vi "Capture and save.vi"() -> ()   [LabVIEW 2023]
uses:
  <vilib>/userDefined/High Color/IMAQdx.ctl
  <vilib>/vision/driver/NI_Vision_Acquisition_Software.lvlib
panel:
  in  "Stop Button":bool
  in  "Save":bool
  out "Appended Path":path
  in  "File Path 2":path
  out "Image":T1(plugin-control)
  in  "Session In":T2
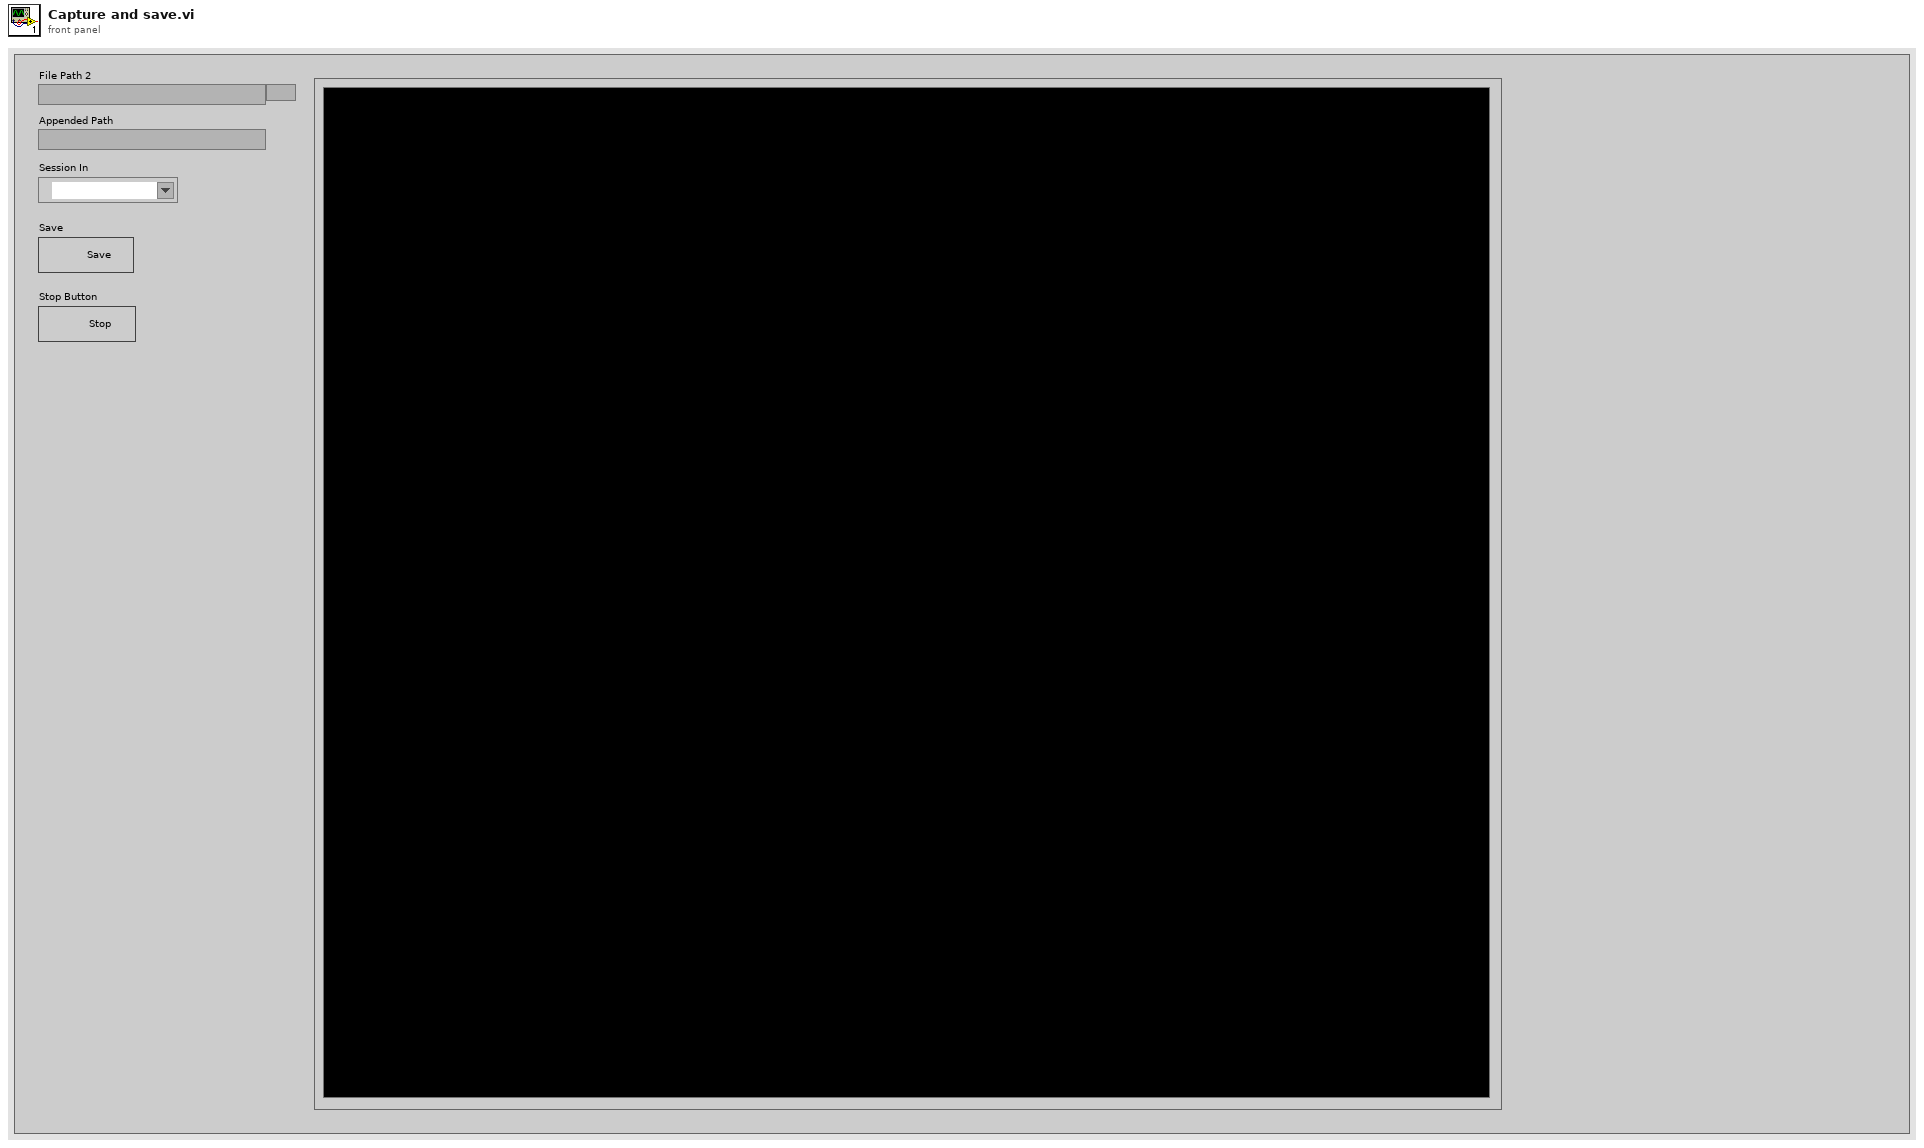
[diagram p1: front panel]
types:
  T1 = typedef "IMAQ Image.ctl" = refnum<image>
  T2 = typedef "IMAQdx.ctl" = refnum<k21>
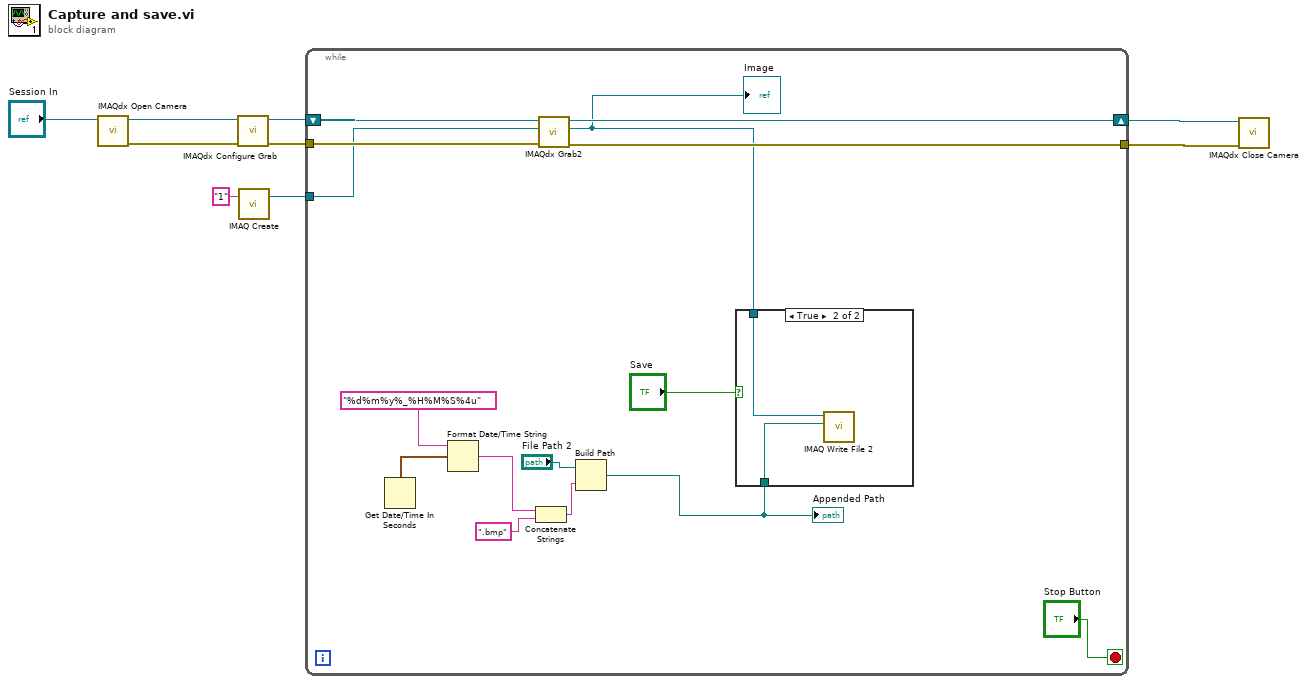
[diagram p0: block diagram]
diagram:
  n1 = call <vilib>:"IMAQdx Open Camera.vi"("Session In"="Session In") -> ("error out"=w8:errorcluster, "Session Out"=w3:T2)  [unwired: 9 in]
  n2 = call <vilib>:"IMAQdx Configure Grab.vi"("error in"=w8, "Session In"=w3) -> ("error out"=w1:errorcluster, "Session Out"=w2:T2)  [unwired: 8 in]
  n3 = call "IMAQ Create"("Image Name"="1") -> ("New Image"=w4:T1)  [unwired: 4 in, 1 out]
  n4 = while {
    shift-right: [w21] -> w7
    shift-left: w2 -> [w24]
    tunnel: w1 -> [w23]
    tunnel: [w22] -> w6
    tunnel: w4 -> [w20]
    stop <- "Stop Button" stop-if-true
    n5 = Get Date/Time In Seconds() -> (seconds since 1Jan1904=w18:timestamp)
    n6 = Format Date/Time String(time format string (%c)="%d%m%y%_%H%M%S%4u", seconds (now)=w18) -> (date/time string=w19:string)  [unwired: 1 in]
    n7 = Concatenate Strings(w19, ".bmp") -> (w17:string)
    n8 = call <vilib>:"IMAQdx Grab2.vi"("error in"=w23, "Image In"=w20, "Session In"=w24) -> ("error out"=w22:errorcluster, "Image Out"=w12:T1, "Session Out"=w21:T2)  [unwired: 5 in, 1 out]
    "Image" <- w12
    n9 = Build Path(base path="File Path 2", name or relative path=w17) -> (appended path=w16:path)
    "Appended Path" <- w16
    n10 = case shown="True" "Save" {
      tunnel: w16 -> [_ w26]
      tunnel: w12 -> [_ w25]
      frame False {
      }
      frame True {
        n11 = call-poly "IMAQ Write File 2"("File Path"=w26, "Image"=w25) -> ()  [unwired: 8 in, 2 out]
      }
    }
  }
  n12 = call <vilib>:"IMAQdx Close Camera.vi"("error in"=w6, "Session In"=w7) -> ()  [unwired: 9 in, 1 out]
